vi "dfd_Convert Param String to MRate Filter.vi"(8 "error in (no error)":errorcluster, 10 "xml string in":string, 11 "multirate filter in":T1={"mMRate_Structure"=enum."CIC", "mMRate_Mode"=0, "mMRate_Factor"=1, "mMRate_FIRParams"={"mMRate_FIR_H"=[], "mMRate_FIR_IsNyquist?"=FALSE, "mMRate_FIR_IsSymmetric?"=FALSE}, "mMRate_CICParams"={"mMRate_CIC_#Stage"=2, "mMRate_CIC_Lag"=1, "mMRate_CIC_Type"=enum."Lowpass"}, "mMRate_Order"=1, "mMRate_Version"="1.0", "mMRate_Comments"="1.0", "mMRate_RationalFactor"={"mMRate_L"=-1, "mMRate_M"=-1}, "mMRate_Fs"=0.0, "mMRate_Quantized?"=FALSE, "mMRate_QFilterGain"=1.0, "mMRate_CoefWl"=16, "mMRate_Scaling"={"mMRate_ScaleByPowerOf2?"=FALSE, "mMRate_ScaleType"=enum."Time Domain 1-Norm"}, "mMRate_InputWl"=0, "mMRate_OutputWl"=0, "mMRate_OutputMode"=enum."Nearest", "mMRate_MultMode"=enum."Truncated", "mMRate_BitPruning"=FALSE, "mMRate_GainWl"=16, "mMRate_OutputFwl"=0, "mMRate_SumIwl"=0, "mMRate_InputIwl "=16, "mMRate_SumWl"=32, "mMRate_CoefIwl"=0} {"mMRate_SumWl" min=1 max=32 step=1; "mMRate_InputIwl" min=1 max=32 step=1; "mMRate_GainWl" min=1 max=32 step=1; "mMRate_OutputWl" min=1 max=32 step=1; "mMRate_InputWl" min=1 max=32 step=1; "mMRate_CoefWl" min=1 max=32 step=1; "mMRate_Mode" items=["Default"=-1, "No Rate Change"=0, "Interpolation"=1, "Decimation"=2, "Interpolated"=3, "Rational"=4]}) -> (0 "error out":errorcluster, 3 "dup multirate filter":T1={"mMRate_Structure"=enum."FIR", "mMRate_Mode"=0, "mMRate_Factor"=1, "mMRate_FIRParams"={"mMRate_FIR_H"=[], "mMRate_FIR_IsNyquist?"=FALSE, "mMRate_FIR_IsSymmetric?"=FALSE}, "mMRate_CICParams"={"mMRate_CIC_#Stage"=2, "mMRate_CIC_Lag"=1, "mMRate_CIC_Type"=enum."Lowpass"}, "mMRate_Order"=0, "mMRate_Version"="2.0", "mMRate_Comments"="", "mMRate_RationalFactor"={"mMRate_L"=-1, "mMRate_M"=-1}, "mMRate_Fs"=1.0, "mMRate_Quantized?"=FALSE, "mMRate_QFilterGain"=1.0, "mMRate_CoefWl"=16, "mMRate_Scaling"={"mMRate_ScaleByPowerOf2?"=FALSE, "mMRate_ScaleType"=enum."Time Domain 1-Norm"}, "mMRate_InputWl"=16, "mMRate_OutputWl"=16, "mMRate_OutputMode"=enum."Nearest", "mMRate_MultMode"=enum."Truncated", "mMRate_BitPruning"=FALSE, "mMRate_GainWl"=16, "mMRate_OutputFwl"=0, "mMRate_SumIwl"=0, "mMRate_InputIwl "=16, "mMRate_SumWl"=32, "mMRate_CoefIwl"=0} {"mMRate_SumWl" min=1 max=32 step=1; "mMRate_InputIwl" min=1 max=32 step=1; "mMRate_GainWl" min=1 max=32 step=1; "mMRate_OutputWl" min=1 max=32 step=1; "mMRate_InputWl" min=1 max=32 step=1; "mMRate_CoefWl" min=1 max=32 step=1; "mMRate_Mode" items=["Default"=-1, "No Rate Change"=0, "Interpolation"=1, "Decimation"=2, "Interpolated"=3, "Rational"=4]})   [LabVIEW 2017, in "NI_DigFilter_Process.lvlib"]
uses:
  <vilib>/addons/Digital Filter Design/NI_DigFilter_Process.lvlib
  <vilib>/addons/Digital Filter Design/_Objects.llb/DFD Multirate Filter Obj.ctl
  <vilib>/addons/Digital Filter Design/_Objects.llb/DFD Multirate Mode.ctl
  <vilib>/addons/Digital Filter Design/_Objects.llb/DFD Coef Norm Type.ctl
  <vilib>/addons/Digital Filter Design/_Objects.llb/DFD Round-off Mode.ctl
  <vilib>/addons/Digital Filter Design/_Objects.llb/DFD FXP MRate Multiply Mode.ctl
  <vilib>/addons/Digital Filter Design/NI_DigFilterLicensed.lvlib
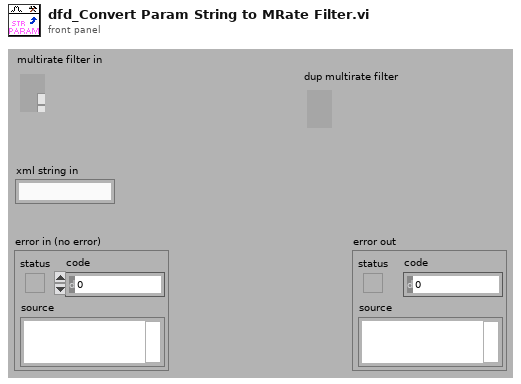
[diagram p1: front panel]
types:
  T1 = typedef "NI_DigFilterLicensed.lvlib/DFD Multirate Filter Obj.ctl" = cluster{"mMRate_Structure":enum16{"CIC", "FIR", "IIR", "Lattice"}, "mMRate_Mode":T2, "mMRate_Factor":i32, "mMRate_FIRParams":cluster{"mMRate_FIR_H":dbl[], "mMRate_FIR_IsNyquist?":bool, "mMRate_FIR_IsSymmetric?":bool}, "mMRate_CICParams":cluster{"mMRate_CIC_#Stage":i32, "mMRate_CIC_Lag":i32, "mMRate_CIC_Type":enum16{"Lowpass", "Highpass"}}, "mMRate_Order":i32, "mMRate_Version":string, "mMRate_Comments":string, "mMRate_RationalFactor":cluster{"mMRate_L":i32, "mMRate_M":i32}, "mMRate_Fs":dbl, "mMRate_Quantized?":bool, "mMRate_QFilterGain":dbl, "mMRate_CoefWl":i16, "mMRate_Scaling":cluster{"mMRate_ScaleByPowerOf2?":bool, "mMRate_ScaleType":T3}, "mMRate_InputWl":i16, "mMRate_OutputWl":i16, "mMRate_OutputMode":T4, "mMRate_MultMode":T5, "mMRate_BitPruning":bool, "mMRate_GainWl":i16, "mMRate_OutputFwl":i16, "mMRate_SumIwl":i16, "mMRate_InputIwl ":i16, "mMRate_SumWl":i16, "mMRate_CoefIwl":i16}
  T2 = typedef "NI_DigFilterLicensed.lvlib/DFD Multirate Mode.ctl" = i16
  T3 = typedef "NI_DigFilterLicensed.lvlib/DFD Coef Norm Type.ctl" = enum16{"No Norm", "Time Domain 1-Norm", "Time Domain 2-Norm", "Time Domain Inf-Norm"}
  T4 = typedef "NI_DigFilterLicensed.lvlib/DFD Round-off Mode.ctl" = enum16{"Nearest", "Truncation"}
  T5 = typedef "NI_DigFilterLicensed.lvlib/DFD FXP MRate Multiply Mode.ctl" = enum16{"Truncated", "Full"}
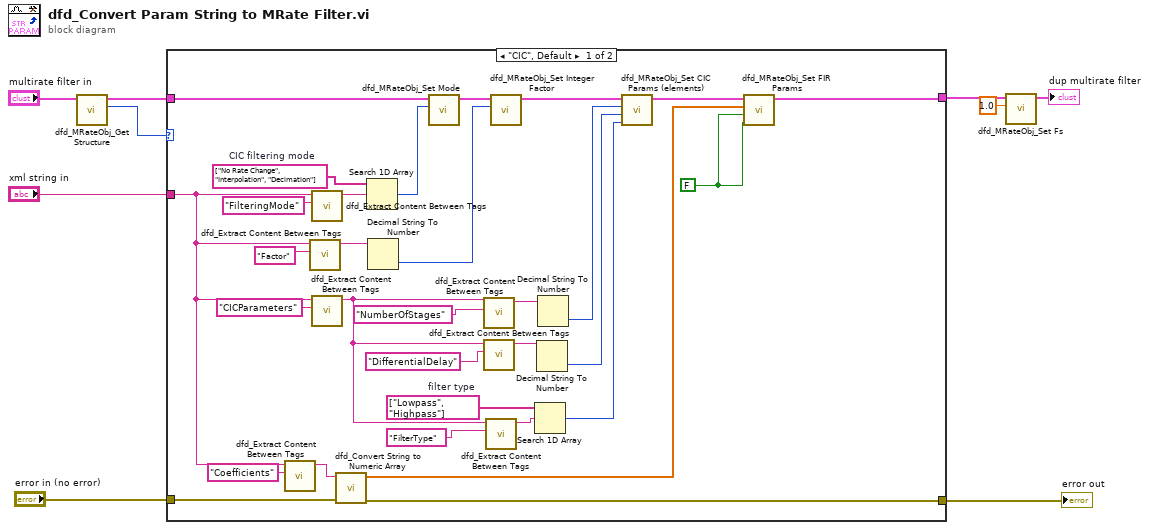
[diagram p0: block diagram]
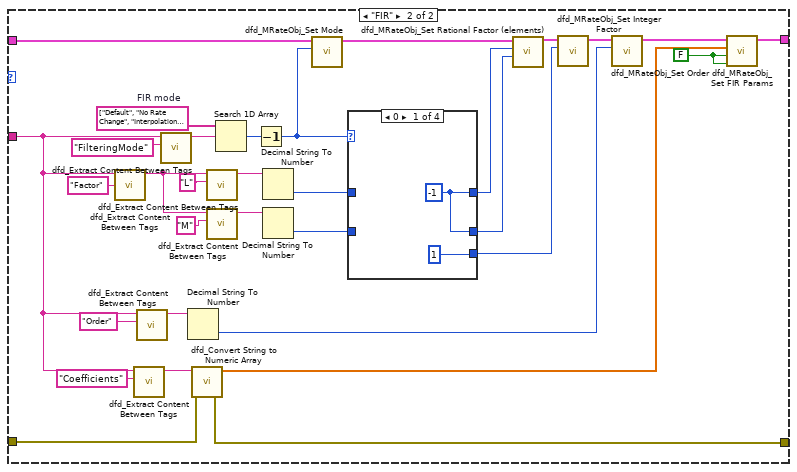
[diagram p2: hidden frame]
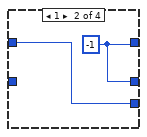
[diagram p3: hidden frame]
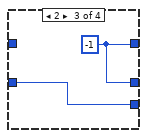
[diagram p4: hidden frame]
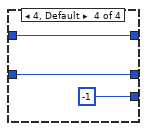
[diagram p5: hidden frame]
diagram:
  n1 = call <vilib>:"dfd_MRateObj_Get Structure.vi"("multirate filter in"="multirate filter in") -> ("structure"=w8:enum16{"CIC", "FIR", "IIR", "Lattice"}, "dup multirate filter"=w6:T1)  [unwired: 9 out]
  n2 = case shown="\"CIC\", Default" w8 {
    tunnel: "xml string in" -> [w30 w58]
    tunnel: w6 -> [w31 w60]
    tunnel: "error in (no error)" -> [w29 w55]
    tunnel: [w14 w52] -> w4
    tunnel: [w13 w51] -> w3
    frame "CIC", Default {
      w10 = string[] ["No Rate Change", "Interpolation", "Decimation"]  # CIC filtering mode
      w11 = string[] ["Lowpass", "Highpass"]  # filter type
      w12 = FALSE ("is Nyquist?")
      n3 = call <vilib>:"dfd_Extract Content Between Tags.vi"("element"="Coefficients", "xml string with tag"=w30) -> ("content"=w32:string)  [unwired: 9 out]
      n4 = call <vilib>:"dfd_Extract Content Between Tags.vi"("element"="Factor", "xml string with tag"=w30) -> ("content"=w28:string)  [unwired: 9 out]
      n5 = call <vilib>:"dfd_Extract Content Between Tags.vi"("element"="FilteringMode", "xml string with tag"=w30) -> ("content"=w39:string)  [unwired: 9 out]
      n6 = call <vilib>:"dfd_Extract Content Between Tags.vi"("element"="CICParameters", "xml string with tag"=w30) -> ("content"=w27:string)  [unwired: 9 out]
      n7 = call <vilib>:"dfd_Convert String to Numeric Array.vi"("error in"=w29, "string"=w32) -> ("error out"=w14:errorcluster, "numeric array"=w15:dbl[])  [unwired: 8 out]
      n8 = Search 1D Array(1D array=w10, element=w39) -> (index of element=w38:i32)  [unwired: 1 out]
      n9 = Decimal String To Number(string=w28) -> (number=w36:i32)  [unwired: 3 out]
      n10 = call <vilib>:"dfd_MRateObj_Set Mode.vi"("mode"=w38, "multirate filter in"=w31) -> ("multirate filter out"=w34:T1)  [unwired: 9 out]
      n11 = call <vilib>:"dfd_Extract Content Between Tags.vi"("element"="NumberOfStages" ("element name"), "xml string with tag"=w27) -> ("content"=w23:string)  [unwired: 9 out]
      n12 = call <vilib>:"dfd_Extract Content Between Tags.vi"("element"="DifferentialDelay" ("element name"), "xml string with tag"=w27) -> ("content"=w22:string)  [unwired: 9 out]
      n13 = call <vilib>:"dfd_Extract Content Between Tags.vi"("element"="FilterType" ("element name"), "xml string with tag"=w27) -> ("content"=w21:string)  [unwired: 9 out]
      n14 = call <vilib>:"dfd_MRateObj_Set Integer Factor.vi"("factor"=w36, "multirate filter in"=w34) -> ("multirate filter out"=w20:T1)  [unwired: 9 out]
      n15 = Search 1D Array(1D array=w11, element=w21) -> (index of element=w17:i32)  [unwired: 1 out]
      n16 = Decimal String To Number(string=w22) -> (number=w18:i32)  [unwired: 3 out]
      n17 = Decimal String To Number(string=w23) -> (number=w19:i32)  [unwired: 3 out]
      n18 = call <vilib>:"dfd_MRateObj_Set CIC Params (elements).vi"("type"=w17, "lag"=w18, "# stages"=w19, "multirate filter in"=w20) -> ("multirate filter out"=w16:T1)  [unwired: 7 out]
      n19 = call <vilib>:"dfd_MRateObj_Set FIR Params.vi"("is symmetric?"=w12, "is Nyquist?"=w12, "h(n)"=w15, "multirate filter in"=w16) -> ("multirate filter out"=w13:T1)  [unwired: 7 out]
    }
    frame "FIR" {
      w41 = string[] ["Default", "No Rate Change", "Interpolation", "Decimation", "Interpolated", "Rational"]  # FIR mode
      w42 = FALSE ("is Nyquist?")
      n20 = call <vilib>:"dfd_Extract Content Between Tags.vi"("element"="Factor", "xml string with tag"=w58) -> ("content"=w50:string)  [unwired: 9 out]
      n21 = call <vilib>:"dfd_Extract Content Between Tags.vi"("element"="Coefficients", "xml string with tag"=w58) -> ("content"=w56:string)  [unwired: 9 out]
      n22 = call <vilib>:"dfd_Extract Content Between Tags.vi"("element"="Order", "xml string with tag"=w58) -> ("content"=w64:string)  [unwired: 9 out]
      n23 = call <vilib>:"dfd_Extract Content Between Tags.vi"("element"="FilteringMode", "xml string with tag"=w58) -> ("content"=w71:string)  [unwired: 9 out]
      n24 = Decimal String To Number(string=w64) -> (number=w61:i32)  [unwired: 3 out]
      n25 = call <vilib>:"dfd_Convert String to Numeric Array.vi"("error in"=w55, "string"=w56) -> ("error out"=w52:errorcluster, "numeric array"=w53:dbl[])  [unwired: 8 out]
      n26 = call <vilib>:"dfd_Extract Content Between Tags.vi"("element"="L", "xml string with tag"=w50) -> ("content"=w67:string)  [unwired: 9 out]
      n27 = call <vilib>:"dfd_Extract Content Between Tags.vi"("element"="M", "xml string with tag"=w50) -> ("content"=w65:string)  [unwired: 9 out]
      n28 = Search 1D Array(1D array=w41, element=w71) -> (index of element=w70:i32)  [unwired: 1 out]
      n29 = Decrement(x=w70) -> (x-1=w49:i32)
      n30 = Decimal String To Number(string=w67) -> (number=w48:i32)  [unwired: 3 out]
      n31 = Decimal String To Number(string=w65) -> (number=w47:i32)  [unwired: 3 out]
      n32 = call <vilib>:"dfd_MRateObj_Set Mode.vi"("mode"=w49, "multirate filter in"=w60) -> ("multirate filter out"=w62:T1)  [unwired: 9 out]
      n33 = case shown="0" w49 {
        tunnel: w48 -> [_ w76 _ w81]
        tunnel: w47 -> [_ _ w78 w80]
        tunnel: [w73 w75 w77 w81] -> w46
        tunnel: [w73 w75 w77 w80] -> w45
        tunnel: [1 w76 w78 -1] -> w43
        frame 0 {
          w73 = -1
        }
        frame 1 {
          w75 = -1
        }
        frame 2 {
          w77 = -1
        }
        frame 4, Default {
        }
      }
      n34 = call <vilib>:"dfd_MRateObj_Set Rational Factor (elements).vi"("M"=w45, "L"=w46, "multirate filter in"=w62) -> ("multirate filter out"=w59:T1)  [unwired: 8 out]
      n35 = call <vilib>:"dfd_MRateObj_Set Integer Factor.vi"("factor"=w43, "multirate filter in"=w59) -> ("multirate filter out"=w44:T1)  [unwired: 9 out]
      n36 = call <vilib>:"dfd_MRateObj_Set Order.vi"("order"=w61, "multirate filter in"=w44) -> ("multirate filter out"=w54:T1)  [unwired: 9 out]
      n37 = call <vilib>:"dfd_MRateObj_Set FIR Params.vi"("is symmetric?"=w42, "is Nyquist?"=w42, "h(n)"=w53, "multirate filter in"=w54) -> ("multirate filter out"=w51:T1)  [unwired: 7 out]
    }
  }
  "error out" <- w4
  n38 = call <vilib>:"dfd_MRateObj_Set Fs.vi"("fs"=1.0, "multirate filter in"=w3) -> ("dup multirate filter"=→"dup multirate filter":T1)  [unwired: 9 out]
